vi "3motorVelCtrl (SubVI).vi"(6 "reset Encoder":bool, 7 "motorPort [M0, M1, M2]":T1[](array[typedef])=[enum."M0", enum."M1", enum."M2"], 8 "error in (no error)":errorcluster, 10 "motorSpeed [M0, M1, M2] (deg/s)":dbl[](array[slide]) scale=-450.0..450.0, 11 "TitanQuad in":refnum<class "TitanQuad.lvclass">) -> (0 "error out":errorcluster, 2 "Enc [M0, M1, M2] (deg)":dbl[](array[numeric]), 3 "TitanQuad out":refnum<class "TitanQuad.lvclass">)   [LabVIEW 2020]
uses:
  <vilib>/CISH Robotics/L4VMX TitanQuad/Motor ID.ctl
  <vilib>/CISH Robotics/L4VMX TitanQuad/TitanQuad.lvclass
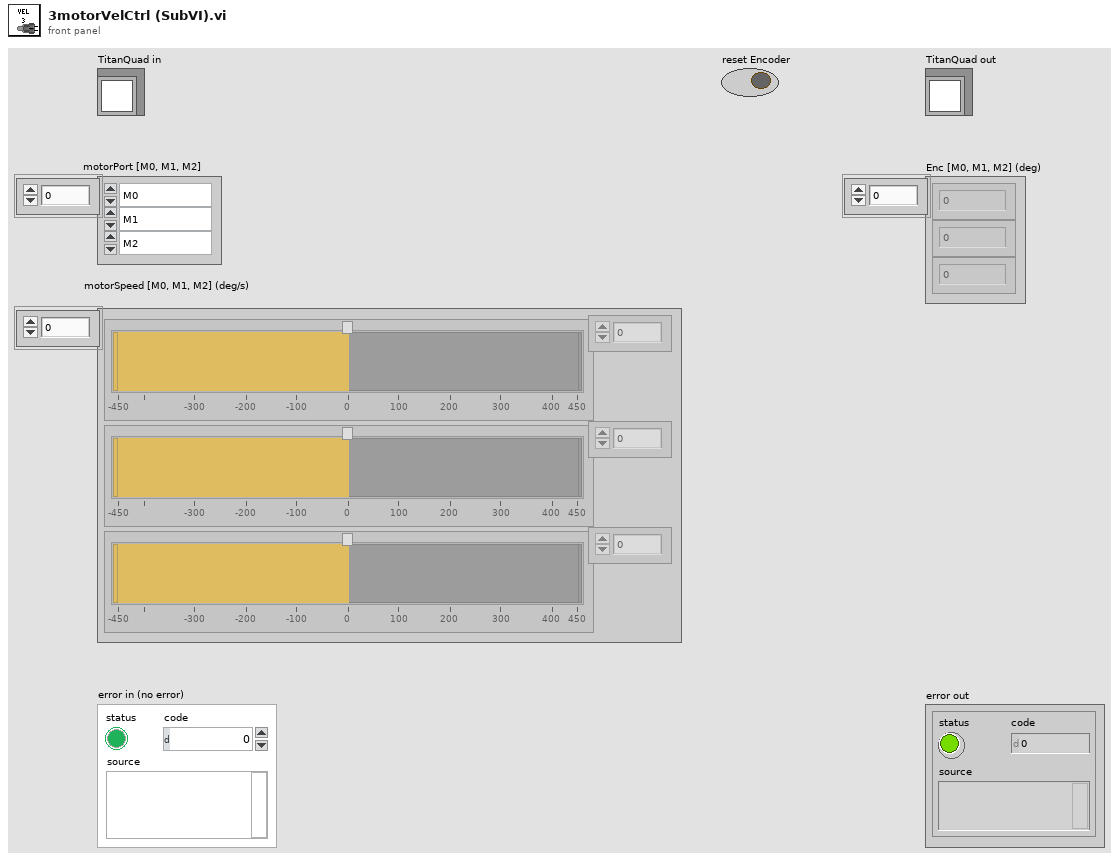
[diagram p1: front panel]
types:
  T1 = typedef "TitanQuad.lvlib/TitanQuad.lvclass/Motor ID.ctl" = enum16{"M0", "M1", "M2", "M3"}
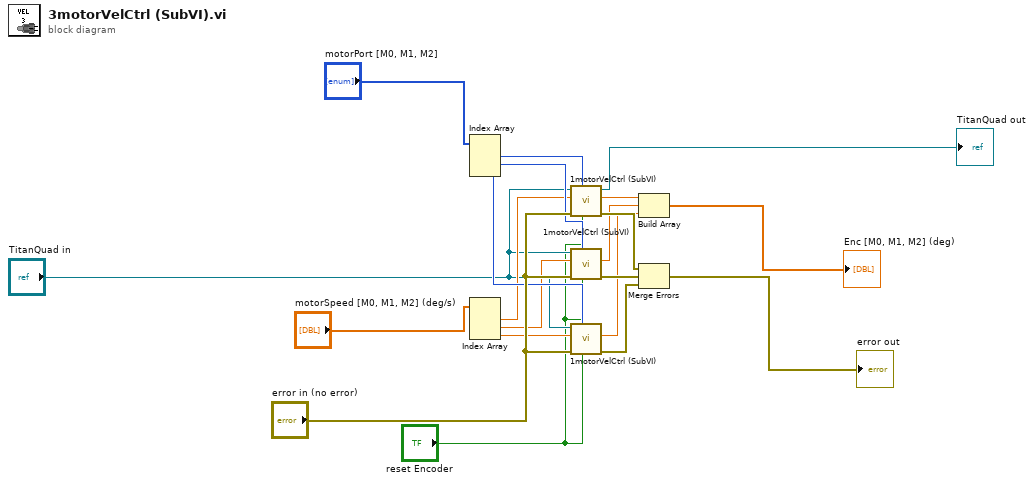
[diagram p0: block diagram]
diagram:
  n1 = Index Array(array="motorPort [M0, M1, M2]") -> (element #1=w9:T1, element #2=w10:T1, element #3=w11:T1)  [unwired: 3 in]
  n2 = Index Array(array="motorSpeed [M0, M1, M2] (deg/s)") -> (element #1=w5:dbl, element #2=w6:dbl, element #3=w7:dbl)  [unwired: 3 in]
  n3 = call "1motorVelCtrl (SubVI).vi"("reset Encoder"="reset Encoder", "Motor ID"=w9, "error in (no error)"="error in (no error)", "motorSpeed (deg/s)"=w5, "TitanQuad in"="TitanQuad in") -> ("error out"=w17:errorcluster, "Enc (deg)"=w13:dbl, "TitanQuad out"=→"TitanQuad out":refnum<class "TitanQuad.lvclass">)  [unwired: 3 in, 1 out]
  n4 = call "1motorVelCtrl (SubVI).vi"("reset Encoder"="reset Encoder", "Motor ID"=w10, "error in (no error)"="error in (no error)", "motorSpeed (deg/s)"=w6, "TitanQuad in"="TitanQuad in") -> ("error out"=w18:errorcluster, "Enc (deg)"=w14:dbl)  [unwired: 3 in, 2 out]
  n5 = call "1motorVelCtrl (SubVI).vi"("reset Encoder"="reset Encoder", "Motor ID"=w11, "error in (no error)"="error in (no error)", "motorSpeed (deg/s)"=w7, "TitanQuad in"="TitanQuad in") -> ("error out"=w19:errorcluster, "Enc (deg)"=w15:dbl)  [unwired: 3 in, 2 out]
  n6 = Build Array(w13, w14, w15) -> (→"Enc [M0, M1, M2] (deg)":dbl[])
  n7 = Merge Errors(w17, w18, w19) -> (→"error out":errorcluster)
